vi "magnet-read.vi"(8 "error in (no error)":errorcluster, 11 "magnet IN":refnum<class "Magnet.lvclass">) -> (0 "error out":errorcluster, 2 "Result":dbl[](array[numeric]), 3 "magnet OUT":refnum<class "Magnet.lvclass">)   [LabVIEW 2018, in "Magnet.lvclass"]
uses:
  Magnet.lvclass
  Users/Shared/github/NHMFL_Core/Libraries/Instruments/Instrument Driver/Instrument Driver.lvclass
  resonant_ultrasound_arxiv/maglab ultrasound -- arkady --arxiv/publisher action.ctl
  NHMFL_Core/Libraries/Instruments/Instrument Driver/Instrument Driver.lvclass/Instrument Driver.ctl
  NHMFL_Core/Libraries/Instruments/Instrument Driver/Write Channel names.vi
  NHMFL_Core/Libraries/Instruments/Instrument Driver/Write Channel units.vi
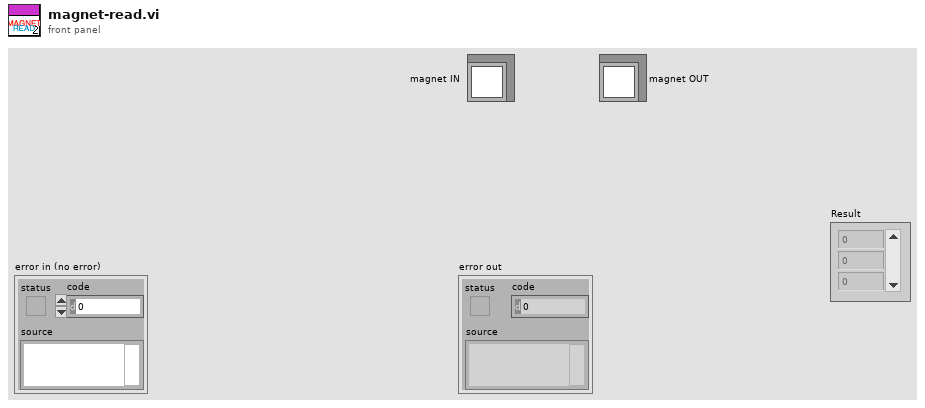
[diagram p1: front panel]
types:
  T1 = typedef "publisher action.ctl" = enum16{"set", "get"}
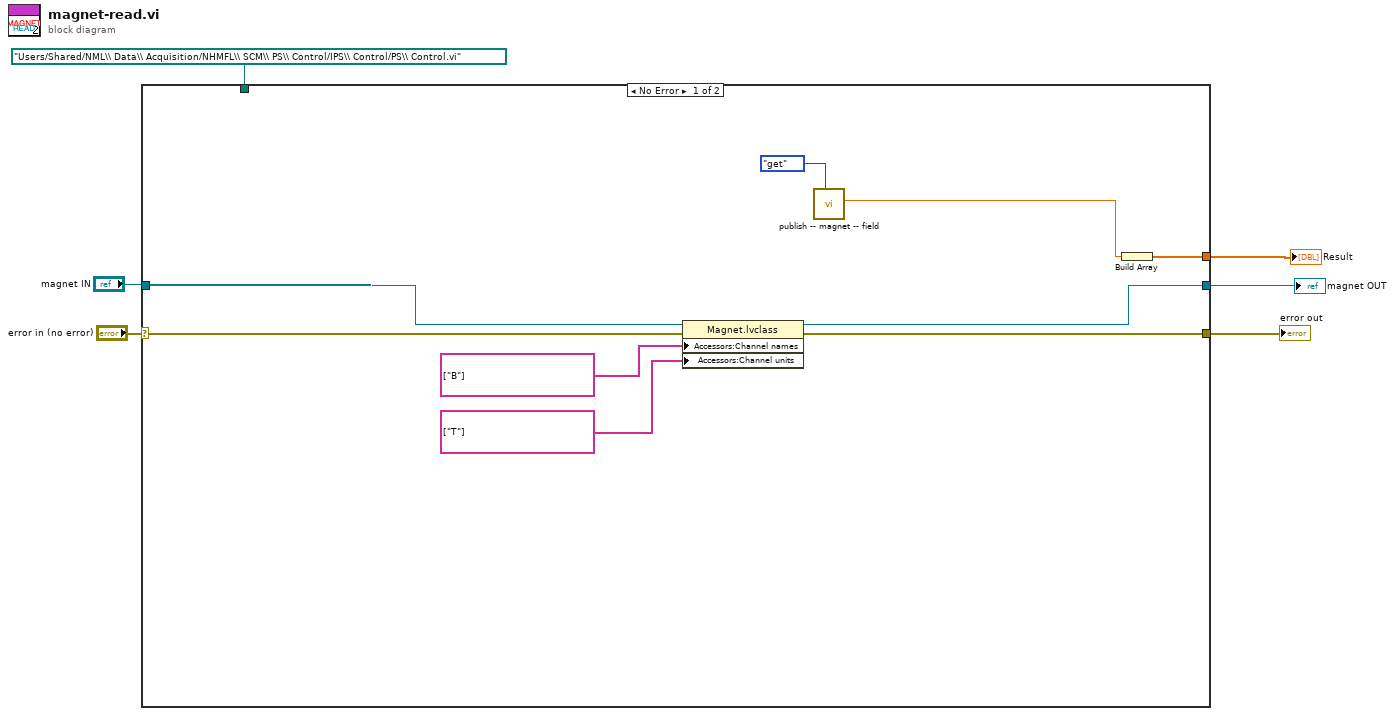
[diagram p0: block diagram]
diagram:
  n1 = case shown="No Error" "error in (no error)" {
    selector: "error in (no error)" -> [w12 w17]
    tunnel: [w9 w17] -> w5
    tunnel: [w13 w16] -> w4
    tunnel: "magnet IN" -> [w14 w16]
    tunnel: [w15 _] -> w1
    tunnel: path "/Users/Shared/NML\\ Data\\ Acquisition/NHMFL\\ SCM\\ PS\\ Control/IPS\\ Control/PS\\ Control.vi" ("vi path") -> [_ _]
    frame No Error {
      n2 = property class="Magnet.lvclass"(reference=w14, error in=w12, "Accessors:Channel names"=string[] ["B"] ("Channel names"), "Accessors:Channel units"=string[] ["T"] ("Channel names")) -> (reference out=w13:refnum<class "Magnet.lvclass">, error out=w9:errorcluster)
      n3 = call "publish -- magnet -- field.vi"("publisher action"=publisher_action."get") -> ("Field out (T)"=w7:dbl)  [unwired: 10 in]
      n4 = Build Array(w7) -> (w15:dbl[])
    }
    frame Error {
    }
  }
  "error out" <- w5
  "Result" <- w1
  "magnet OUT" <- w4
